vi "Client.vi"() -> ()   [LabVIEW 2015]
uses:
  SubVIs/Client state.ctl
  SubVIs/Client data.ctl
panel:
  in  "Message":string
  in  "Send":bool
  in  "IP Address":string
  out "Connection":bool
  in  "stop":bool
  in  "port":u16
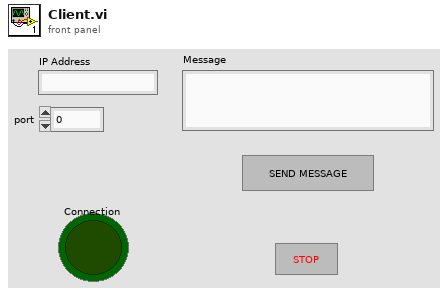
[diagram p1: front panel]
types:
  T1 = typedef "Client data.ctl" = cluster{"connection ID":refnum<k5>, "error IO":errorcluster, "Connection":bool}
  T2 = typedef "Client state.ctl" = enum16{"Init", "Connect", "Write", "Disconnect"}
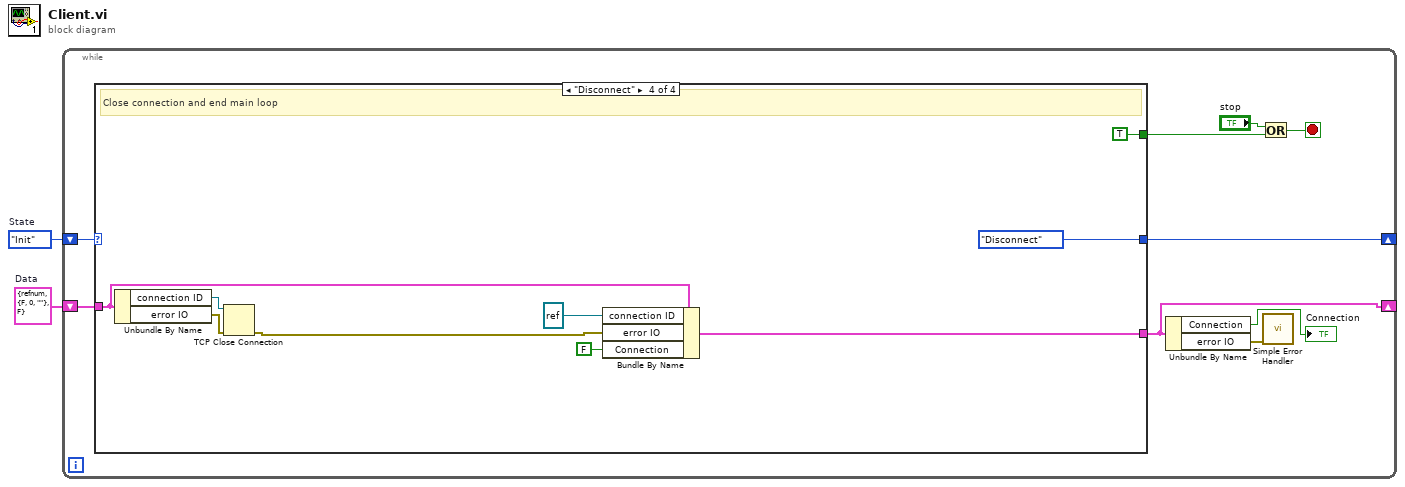
[diagram p0: block diagram]
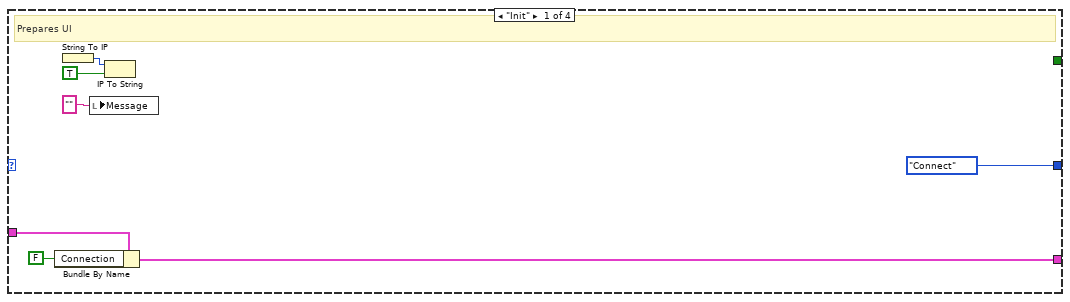
[diagram p2: hidden frame]
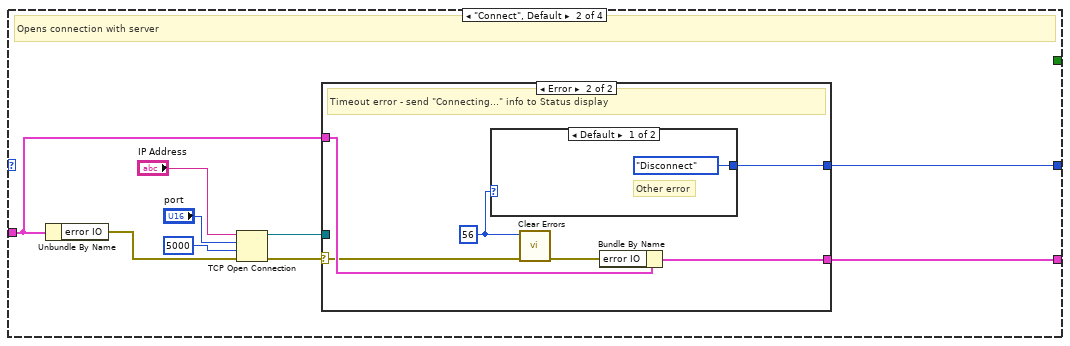
[diagram p3: hidden frame]
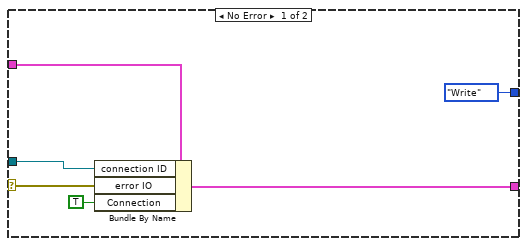
[diagram p4: hidden frame]
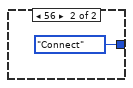
[diagram p5: hidden frame]
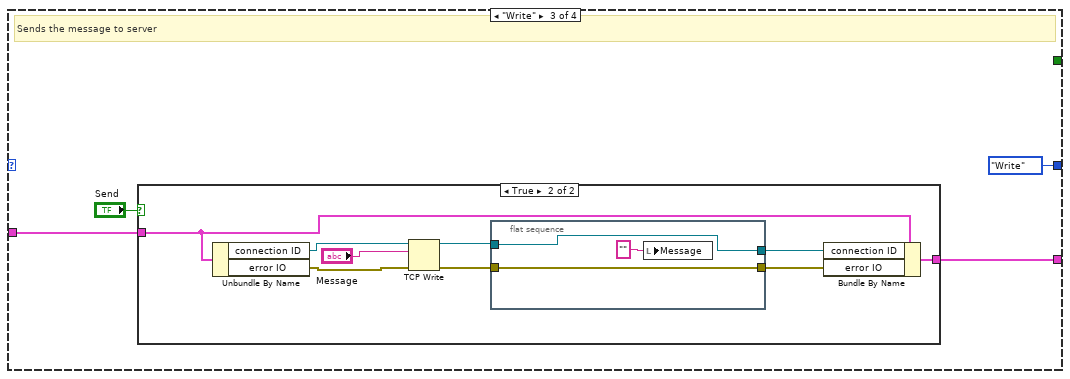
[diagram p6: hidden frame]
diagram:
  w1 = T1 {"connection ID"=refnum, "error IO"={"status"=FALSE, "code"=0, "source"=""}, "Connection"=FALSE}  # Data
  w2 = Client_state."Init"  # State
  n1 = while {
    shift-right: [w9] -> _
    shift-left: w2 -> [w11]
    shift-right: [w7] -> _
    shift-left: w1 -> [w10]
    stop <- w4 stop-if-true
    n2 = case shown="\"Disconnect\"" w11 {
      tunnel: w10 -> [w18 w25 w45 w65]
      tunnel: [w17 w27 w44 w60] -> w7
      tunnel: [Client_state."Connect" ("Enum") w26 Client_state."Write" ("Enum") Client_state."Disconnect" ("Enum")] -> w9
      tunnel: [_ _ _ TRUE ("stop")] -> w5
      frame "Init" {
        # "Prepares UI"
        n3 = Bundle By Name(cluster=w18, "Connection"=FALSE) -> (w17:T1)
        n4 = String To IP() -> (0:w14:u32)  [unwired: 1 in]
        n5 = local write "Message"("" ("Message")) -> ()
        n6 = IP To String(1:TRUE ("dot notation? (F)"), 2:w14) -> ()  [unwired: 1 out]
      }
      frame "Connect", Default {
        # "Opens connection with server"
        n7 = Unbundle By Name(w25) -> ("error IO"=w24:errorcluster)
        n8 = TCP Open Connection(address="IP Address", remote port or service name="port", timeout ms (60000)=5000 ("timeout ms (wait forever: -1)"), error in (no error)=w24) -> (connection ID=w22:refnum<k5>, error out=w23:errorcluster)  [unwired: 1 in]
        n9 = case shown="Error" w23 {
          selector: w23 -> [w28 w37]
          tunnel: w22 -> [w29 _]
          tunnel: w25 -> [w33 w39]
          tunnel: [w31 w38] -> w27
          tunnel: [Client_state."Write" ("Enum") w35] -> w26
          frame No Error {
            n10 = Bundle By Name(cluster=w33, "connection ID"=w29, "error IO"=w28, "Connection"=TRUE) -> (w31:T1)
          }
          frame Error {
            w36 = 56 ("specific error code to clear (0: all)")
            # "Timeout error - send \"Connecting...\" info to Status display"
            n11 = case shown="Default" w36 {
              tunnel: [Client_state."Disconnect" ("Enum") Client_state."Connect" ("Enum")] -> w35
              frame Default {
                # "Other error"
              }
              frame 56 {
              }
            }
            n12 = call <vilib>:"Clear Errors.vi"("error in (no error)"=w37, "specific error code to clear (0: all)"=w36) -> ("error out"=w34:errorcluster)  [unwired: 4 in, 1 out]
            n13 = Bundle By Name(cluster=w39, "error IO"=w34) -> (w38:T1)
          }
        }
      }
      frame "Write" {
        # "Sends the message to server"
        n14 = case shown="True" "Send" {
          tunnel: w45 -> [w46 w54]
          tunnel: [w46 w55] -> w44
          frame False {
          }
          frame True {
            n15 = Unbundle By Name(w54) -> ("connection ID"=w53:refnum<k5>, "error IO"=w52:errorcluster)
            n16 = TCP Write(connection ID=w53, data in="Message", error in (no error)=w52) -> (connection ID out=w49:refnum<k5>, error out=w50:errorcluster)  [unwired: 1 in, 1 out]
            n17 = flat-sequence {
              tunnel: w50 -> [w57]
              tunnel: w49 -> [w58]
              tunnel: [w58] -> w48
              tunnel: [w57] -> w47
              frame #0 {
                n18 = local write "Message"("" ("Message")) -> ()
              }
            }
            n19 = Bundle By Name(cluster=w54, "connection ID"=w48, "error IO"=w47) -> (w55:T1)
          }
        }
      }
      frame "Disconnect" {
        # "Close connection and end main loop"
        n20 = Unbundle By Name(w65) -> ("connection ID"=w67:refnum<k5>, "error IO"=w66:errorcluster)
        n21 = TCP Close Connection(connection ID=w67, error in (no error)=w66) -> (error out=w64:errorcluster)  [unwired: 1 in, 1 out]
        n22 = Bundle By Name(cluster=w65, "connection ID"=refnum<k5> refnum, "error IO"=w64, "Connection"=FALSE) -> (w60:T1)
      }
    }
    n23 = Unbundle By Name(w7) -> ("Connection"=→"Connection":bool, "error IO"=w3:errorcluster)
    n24 = Or(x="stop", y=w5) -> (x .or. y?=w4:bool)
    n25 = call <vilib>:"Simple Error Handler.vi"("error in (no error)"=w3) -> ()  [unwired: 4 in, 5 out]
  }
